vi "Sub_truncate_for_memory.vi"(5 "ACC m/s2":dbl[](array[numeric]), 10 "Experimental Results":T1, 11 "Buffer seconds":i32=60) -> (4 "ACC m/s2":dbl[](array[numeric]))   [LabVIEW 2021]
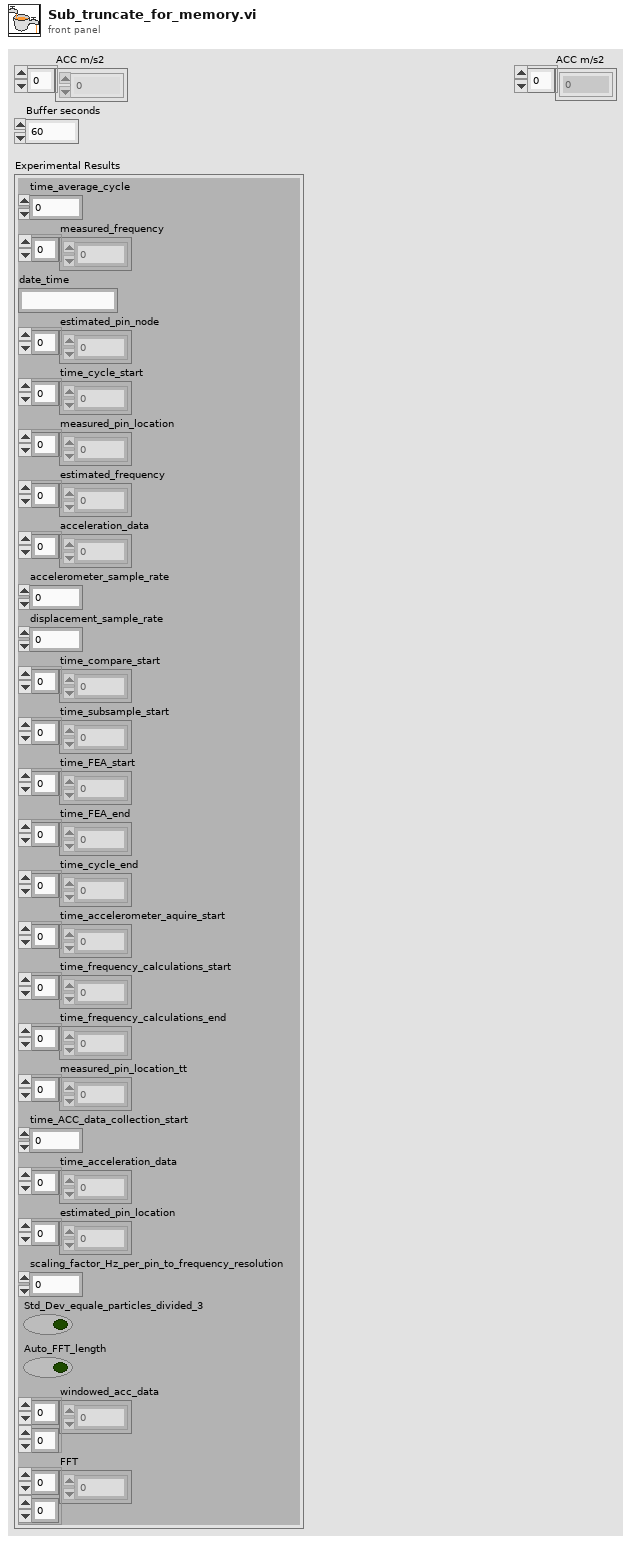
[diagram p1: front panel]
types:
  T1 = cluster{"time_average_cycle":dbl, "measured_frequency":dbl[], "date_time":string, "estimated_pin_node":i32[], "time_cycle_start":dbl[], "measured_pin_location":dbl[], "estimated_frequency":dbl[], "acceleration_data":dbl[], "accelerometer_sample_rate":dbl, "displacement_sample_rate":dbl, "time_compare_start":dbl[], "time_subsample_start":dbl[], "time_FEA_start":dbl[], "time_FEA_end":dbl[], "time_cycle_end":dbl[], "time_accelerometer_aquire_start":dbl[], "time_frequency_calculations_start":dbl[], "time_frequency_calculations_end":dbl[], "measured_pin_location_tt":dbl[], "time_ACC_data_collection_start":dbl, "time_acceleration_data":dbl[], "estimated_pin_location":dbl[], "scaling_factor_Hz_per_pin_to_frequency_resolution":dbl, "Std_Dev_equale_particles_divided_3":bool, "Auto_FFT_length":bool, "windowed_acc_data":dbl[][], "FFT":dbl[][]}
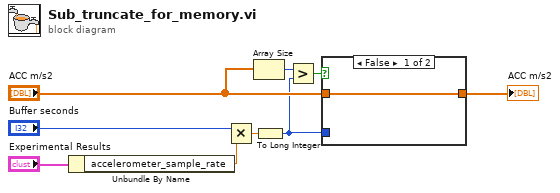
[diagram p0: block diagram]
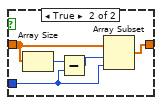
[diagram p2: hidden frame]
diagram:
  n1 = Unbundle By Name("Experimental Results") -> ("accelerometer_sample_rate"=w5:dbl)
  n2 = Multiply(x="Buffer seconds", y=w5) -> (x*y=w4:dbl)
  n3 = Array Size(array="ACC m/s2") -> (size(s)=w9:i32)
  n4 = To Long Integer(number=w4) -> (32bit integer=w1:i32)
  n5 = Greater?(x=w9, y=w1) -> (0:w8:bool)
  n6 = case shown="False" w8 {
    tunnel: w1 -> [_ w12]
    tunnel: "ACC m/s2" -> [w10 w15]
    tunnel: [w10 w11] -> w2
    frame False {
    }
    frame True {
      n7 = Array Size(array=w15) -> (size(s)=w14:i32)
      n8 = Subtract(x=w14, y=w12) -> (x-y=w13:i32)
      n9 = Array Subset(array=w15, index=w13, length=w12) -> (w11:dbl[])
    }
  }
  "ACC m/s2" <- w2
